vi "save 2 file.vi"(8 "error in (no error)":errorcluster, 10 "raw_PDW":u64[][](array[numeric]), 11 "device_type in":refnum<class "device_type.lvclass">) -> (0 "error out":errorcluster, 3 "device_type out":refnum<class "device_type.lvclass">)   [LabVIEW 2021, in "device_type.lvclass"]
uses:
  device_type.lvclass
  device_type.lvclass/device_type.ctl
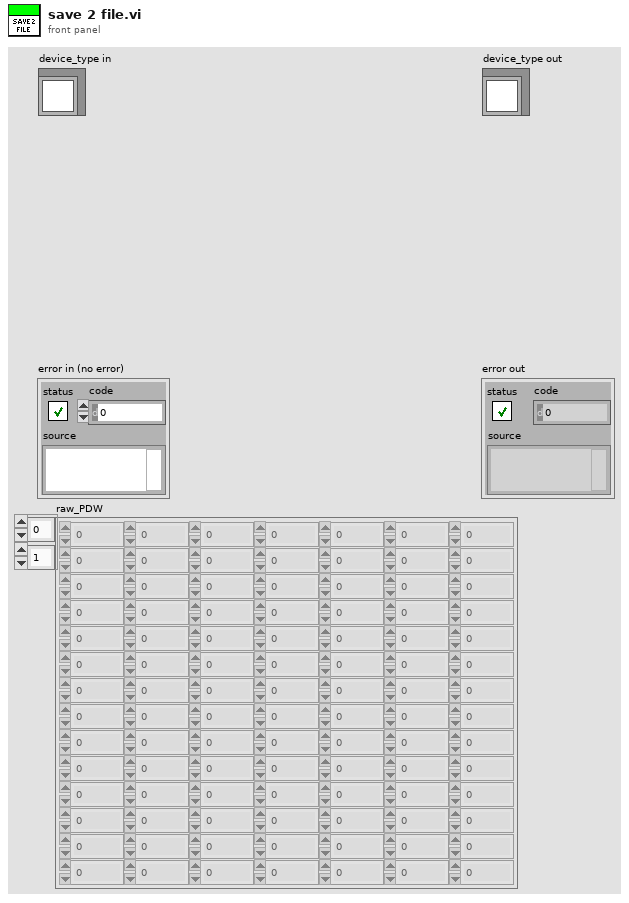
[diagram p1: front panel]
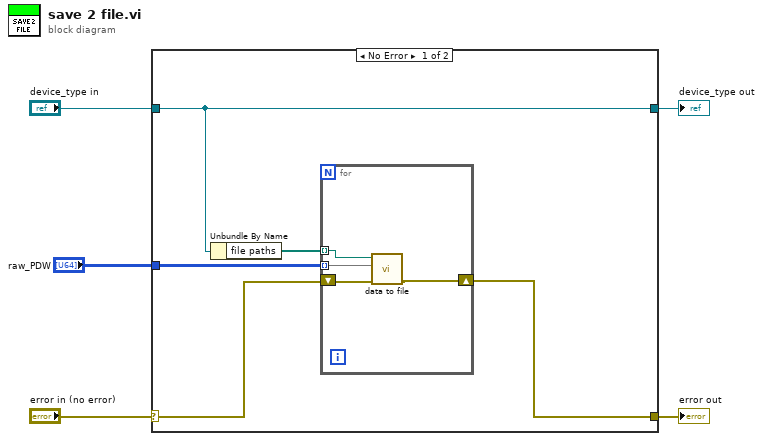
[diagram p0: block diagram]
diagram:
  n1 = case shown="No Error" "error in (no error)" {
    selector: "error in (no error)" -> [w8 w16]
    tunnel: [w6 w16] -> w4
    tunnel: [w7 w15] -> w2
    tunnel: "device_type in" -> [w7 w15]
    tunnel: "raw_PDW" -> [w10 _]
    frame No Error {
      n2 = Unbundle By Name(w7) -> ("file paths"=w9:path[])
      n3 = for {
        tunnel: w10 -> [w14] mode=indexing
        tunnel: w9 -> [w13] mode=indexing
        shift-right: [w11] -> w6
        shift-left: w8 -> [w12]
        n4 = call "data to file.vi"("error in (no error)"=w12, "Array"=w14, "Path"=w13) -> ("error out"=w11:errorcluster)  [unwired: 8 in]
      }
    }
    frame Error {
    }
  }
  "error out" <- w4
  "device_type out" <- w2
